vi "Controller Fast Command Loop.vi"(7 "Sync Objects":T1, 8 "error in (no error)":errorcluster, 11 "FOFB Configuration":T4={"FOFB Parameters"={"Network"={"FOFB Controller IP"="", "LNLS Control Network IP"="", "LNLS Control Network Power Supplies TCP Port"=0, "LNLS Control Network FOFB Configuration TCP Port"=0, "LNLS Control Network BPMs TCP Port"=0, "Monitoring Data TCP Port"=0, "Fast Archiver TCP Port"=0, "Fast Command TCP Port"=0, "TCP Listening Timeout"=0}, "Fast Acquisition"={"Sampling Period"=0, "Data Buffer Size"=0, "Monitoring Period"=0}, "Acquisition Network"=[], "Actuation Network"=[]}, "Number of Acquisition Chassis"=0, "Number of Actuation Chassis"=0, "Number of BPM Readings"=0, "BPM Reading Names"=[], "Selected BPM Readings"=[0, 1, 2, 3, 4, 5, 6, 7, 8, 9, 10, 11, 12, 13, 14, 15, 16, 17, 18, 19, 20, 21, 22, 23, 24, 25, 26, 27, 28, 29, 30, 31, 32, 33, 34, 35, 36, 37, 38, 39, 40, 41, 42, 43, 44, 45, 46, 47, 48, 49], "Number of Correctors"=0, "Corrector Names"=[], "Selected Correctors"=[0, 1, 2, 3, 4, 5, 6, 7, 8, 9, 10, 11, 12, 13, 14, 15, 16, 17, 18, 19, 20, 21, 22, 23, 24, 25, 26, 27, 28, 29, 30, 31, 32, 33, 34, 35, 36, 37, 38, 39, 40, 41, 42, 43, 44, 45, 46, 47, 48, 49], "Response Matrix"=[], "Reference Orbit"=[], "Correction Matrix"=[], "FPGA Filter Sets"=[], "Acquisition Chassis Names"=[], "Actuation Chassis Names"=[], "Acquisition Variables"=[], "Actuation Variables"=[], "PS Matrix Mapping"=[], "Inverse PS Matrix Mapping"=[], "BPM Matrix Mapping"=[], "Inverse BPM Matrix Mapping"=[], "BPM Planes"=[], "Corrector Planes"=[]}) -> (0 "error out":errorcluster)   [LabVIEW 2011]
uses:
  Types Definitions/Type FOFB Configuration.ctl
  Types Definitions/Type FOFB Parameters.ctl
  Types Definitions/Type Network Configuration.ctl
  Types Definitions/Type FA Configuration.ctl
  Types Definitions/Type Acquisition Network Configuration.ctl
  Types Definitions/Type Actuation Network Configuration.ctl
  Types Definitions/Type Synchronization Objects.ctl
  Types Definitions/Type Blocking Synchronization Objects.ctl
  Types Definitions/Type Monitoring Data.ctl
  Types Definitions/Type Operation Mode State.ctl
  Types Definitions/Type Diagnostics Data.ctl
  Types Definitions/Type CPU Loads Array.ctl
  Types Definitions/Type CPU Loads.ctl
  Types Definitions/Type Non-blocking Synchronization Objects.ctl
  Types Definitions/Type FOFB Variables.ctl
  Types Definitions/Type Actuation State.ctl
  Types Definitions/Type TCP State.ctl
  <vilib>/Platform/TimedLoop/XDataNode/timing_clust.ctl
  <vilib>/Platform/TimedLoop/XDataNode/nitl_modes.ctl
  <vilib>/Platform/TimedLoop/XDataNode/wakeup.ctl
  <vilib>/Platform/TimedLoop/XDataNode/XDataNode.xnode
  Type Definitions.lvlib
  <vilib>/Platform/TimedLoop/XDataNode/XDNodeRunTimeDep.lvlib
  Misc VIs.lvlib
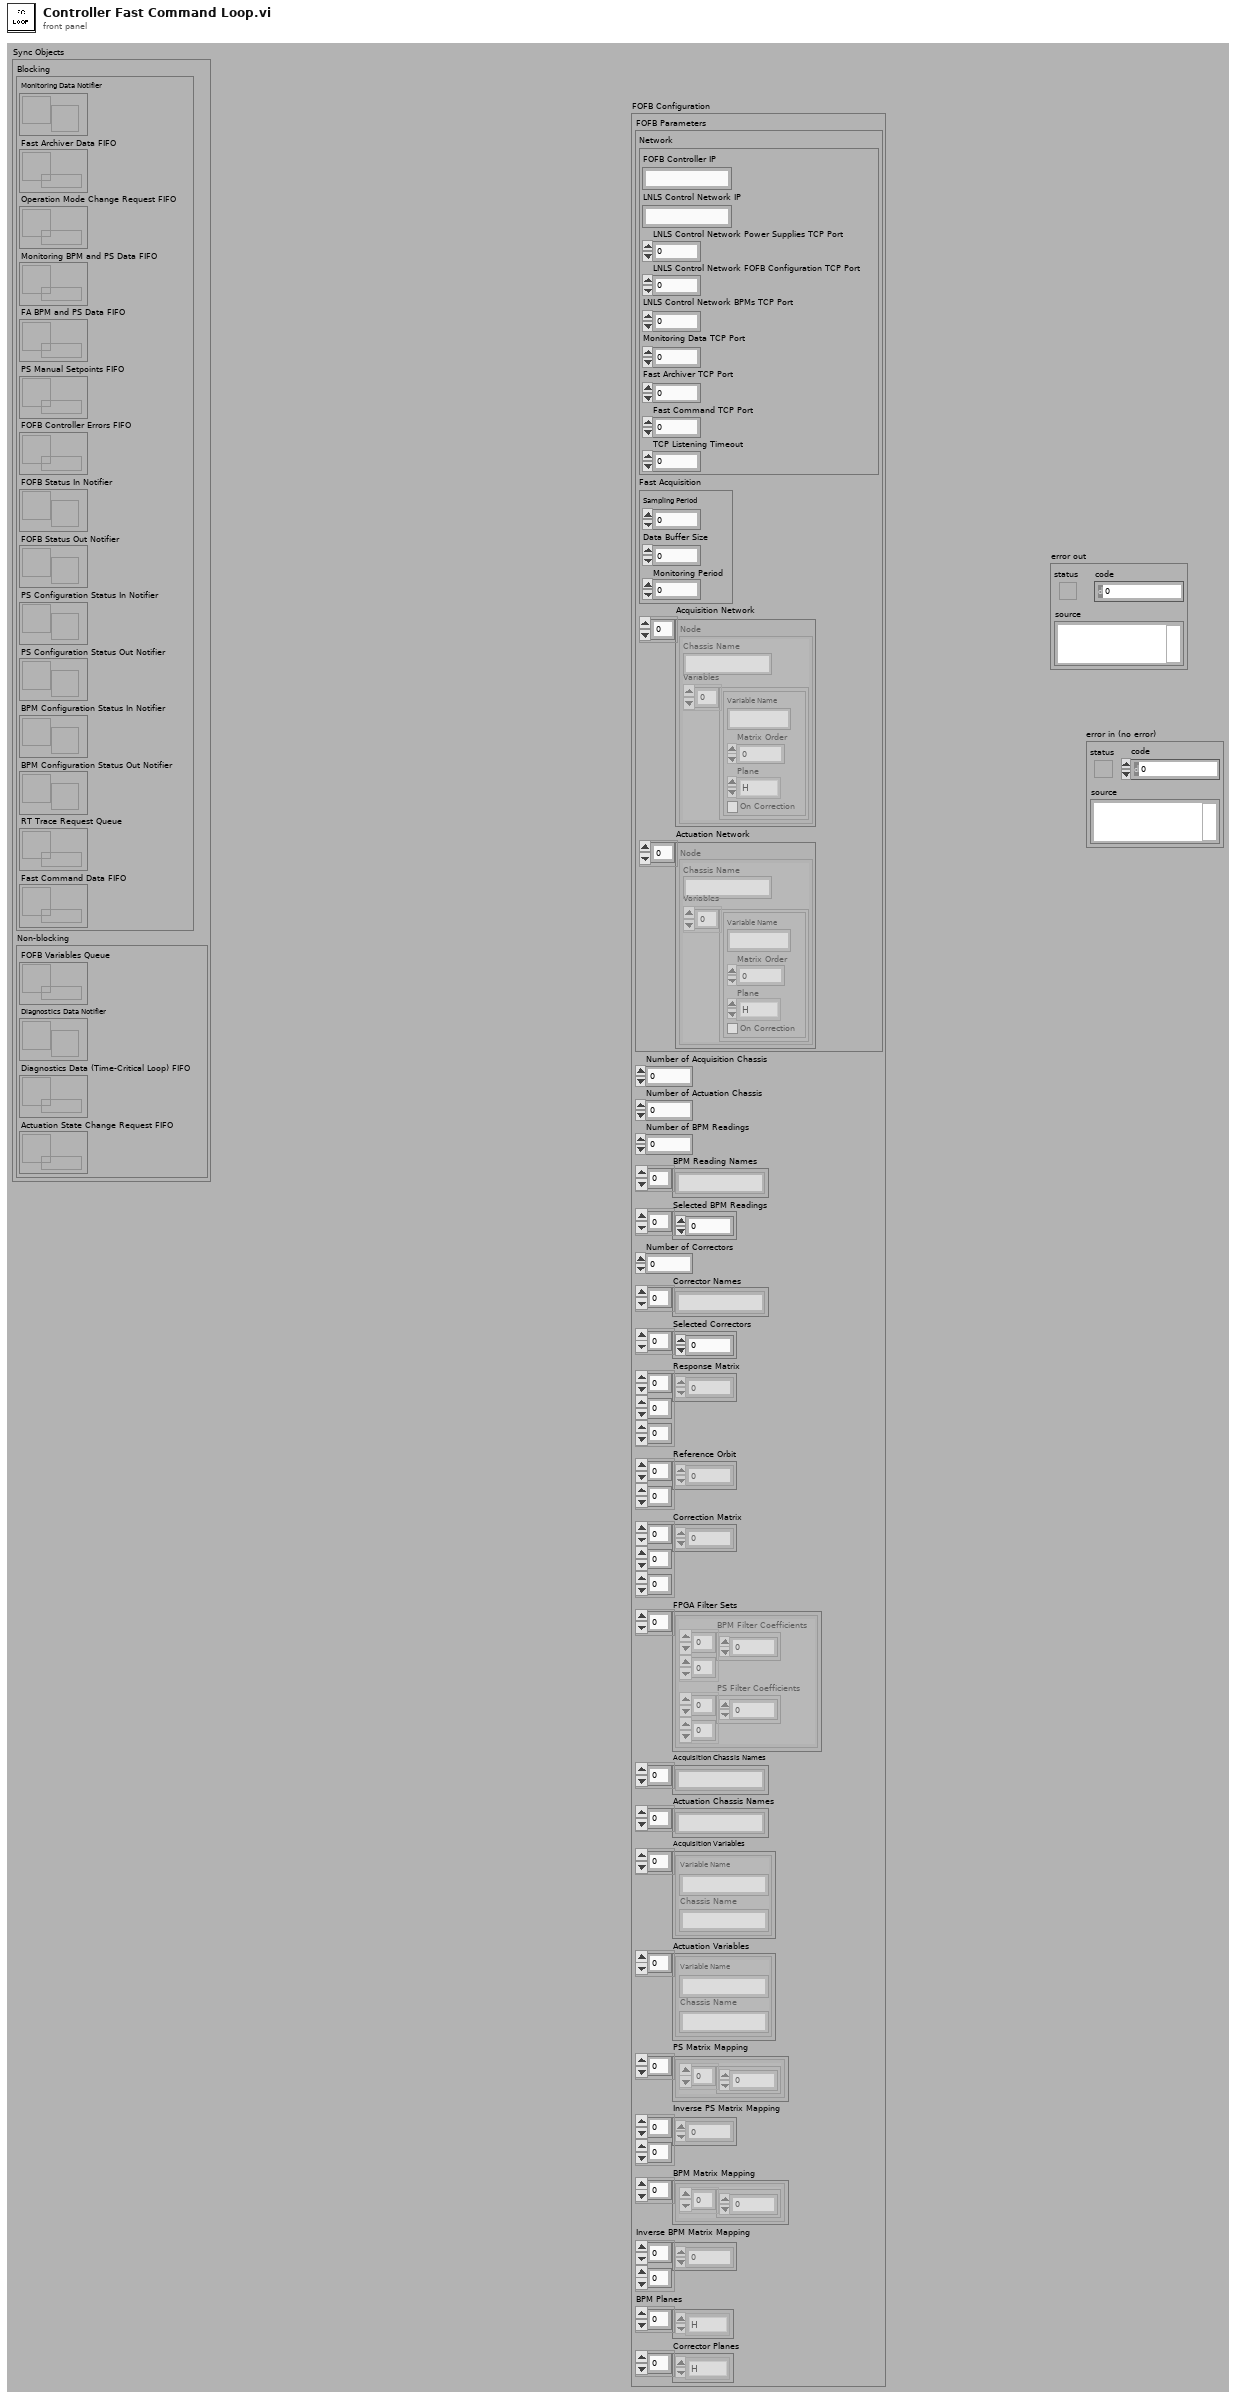
[diagram p1: front panel]
types:
  T1 = typedef "Type Definitions.lvlib/Type Synchronization Objects.ctl" = cluster{"Blocking":T2, "Non-blocking":T3}
  T2 = typedef "Type Definitions.lvlib/Type Blocking Synchronization Objects.ctl" = cluster{"Monitoring Data Notifier":refnum<notifier>, "Fast Archiver Data FIFO":refnum<queue>, "Operation Mode Change Request FIFO":refnum<k33>, "Monitoring BPM and PS Data FIFO":refnum<k33>, "FA BPM and PS Data FIFO":refnum<k33>, "PS Manual Setpoints FIFO":refnum<k33>, "FOFB Controller Errors FIFO ":refnum<k33>, "FOFB Status In Notifier":refnum<notifier>, "FOFB Status Out Notifier":refnum<notifier>, "PS Configuration Status In Notifier":refnum<notifier>, "PS Configuration Status Out Notifier":refnum<notifier>, "BPM Configuration Status In Notifier":refnum<notifier>, "BPM Configuration Status Out Notifier":refnum<notifier>, "RT Trace Request Queue":refnum<queue>, "Fast Command Data FIFO":refnum<k33>}
  T3 = typedef "Type Definitions.lvlib/Type Non-blocking Synchronization Objects.ctl" = cluster{"FOFB Variables Queue":refnum<queue>, "Diagnostics Data Notifier":refnum<notifier>, "Diagnostics Data (Time-Critical Loop) FIFO":refnum<k33>, "Actuation State Change Request FIFO":refnum<k33>}
  T4 = typedef "Type Definitions.lvlib/Type FOFB Configuration.ctl" = cluster{"FOFB Parameters":T5, "Number of Acquisition Chassis":i32, "Number of Actuation Chassis":i32, "Number of BPM Readings":i32, "BPM Reading Names":string[], "Selected BPM Readings":u32[], "Number of Correctors":i32, "Corrector Names":string[], "Selected Correctors":u32[], "Response Matrix":dbl[][][], "Reference Orbit":dbl[][], "Correction Matrix":dbl[][][], "FPGA Filter Sets":cluster{"BPM Filter Coefficients":dbl[][], "PS Filter Coefficients":dbl[][]}[], "Acquisition Chassis Names":string[], "Actuation Chassis Names":string[], "Acquisition Variables":cluster{"Variable Name":string, "Chassis Name":string}[], "Actuation Variables":cluster{"Variable Name":string, "Chassis Name":string}[], "PS Matrix Mapping":cluster{u32[]}[], "Inverse PS Matrix Mapping":u32[][], "BPM Matrix Mapping":cluster{u32[]}[], "Inverse BPM Matrix Mapping":u32[][], "BPM Planes":enum8{"H", "V"}[], "Corrector Planes":enum8{"H", "V"}[]}
  T5 = typedef "Type Definitions.lvlib/Type FOFB Parameters.ctl" = cluster{"Network":T6, "Fast Acquisition":T7, "Acquisition Network":T8, "Actuation Network":T9}
  T6 = typedef "Type Definitions.lvlib/Type Network Configuration.ctl" = cluster{"FOFB Controller IP":string, "LNLS Control Network IP":string, "LNLS Control Network Power Supplies TCP Port":u16, "LNLS Control Network FOFB Configuration TCP Port":u16, "LNLS Control Network BPMs TCP Port":u16, "Monitoring Data TCP Port":u16, "Fast Archiver TCP Port":u16, "Fast Command TCP Port":u16, "TCP Listening Timeout":i32}
  T7 = typedef "Type Definitions.lvlib/Type FA Configuration.ctl" = cluster{"Sampling Period":u32, "Data Buffer Size":u32, "Monitoring Period":u32}
  T8 = typedef "Type Definitions.lvlib/Type Acquisition Network Configuration.ctl" = cluster{"Chassis Name":string, "Variables":cluster{"Variable Name":string, "Matrix Order":u32, "Plane":enum8{"H", "V"}, "On Correction":bool}[]}[]
  T9 = typedef "Type Definitions.lvlib/Type Actuation Network Configuration.ctl" = cluster{"Chassis Name":string, "Variables":cluster{"Variable Name":string, "Matrix Order":u32, "Plane":enum8{"H", "V"}, "On Correction":bool}[]}[]
  T10 = enum16{"big-endian, network order", "native, host order", "little-endian"}
  T11 = typedef "Type Definitions.lvlib/Type TCP State.ctl" = enum16{"Idle", "Wait Connection", "Read Data", "Process Data", "Write Data", "Close Connection"}
  T12 = typedef "XDNodeRunTimeDep.lvlib/timing_clust.ctl" = cluster{"Expected End [f-1]":u64, "Actual End [f-1]":u64, "Finished Late? [f-1]":bool, "Expected End [i-1]":u64, "Actual End [i-1]":u64, "Finished Late? [i-1]":bool, "Expected Start [i]":u64, "Actual Start [i]":u64, "Expected Start [f]":u64, "Actual Start [f]":u64, "Source Name":string, "Structure Name":string, "Period":i64, "Deadline":i64, "Offset":i64, "Start":i64, "Priority":i32, "Timeout":i32, "Mode":T13, "Wakeup Reason":T14, "Error":errorcluster, "Source Type":string, "Secondary Source Type":string, "Global End Time":u64, "Global Start Time":u64, "Frame Duration":u64, "Iteration Duration":u64, "Assigned CPU":i32, "I/O Scan Engine Mode":u32}
  T13 = typedef "XDNodeRunTimeDep.lvlib/nitl_modes.ctl" = enum32{"No Change", "Process missed periods, maintain original phase", "Discard missed periods, maintain original phase", "Process missed periods, ignore original phase", "Discard missed periods, ignore original phase"}
  T14 = typedef "XDNodeRunTimeDep.lvlib/wakeup.ctl" = enum32{"Normal", "Aborted", "Asynchronous wakeup", "Timing source error", "Timed loop error", "Timeout"}
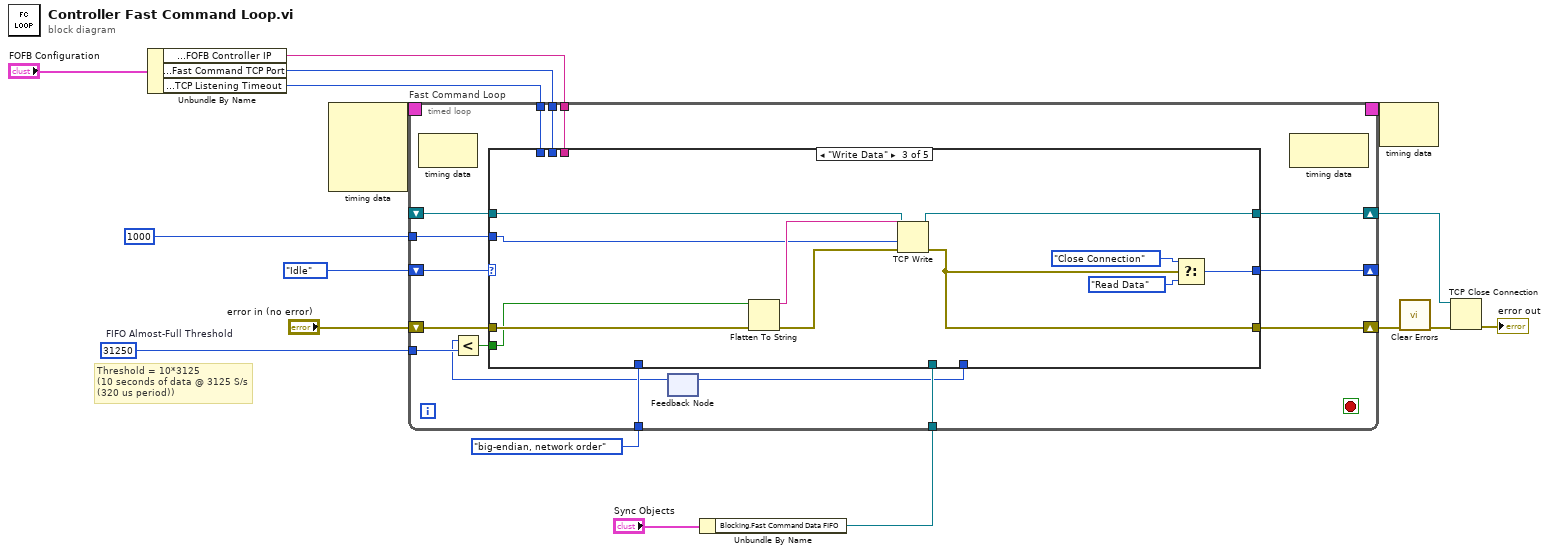
[diagram p0: block diagram]
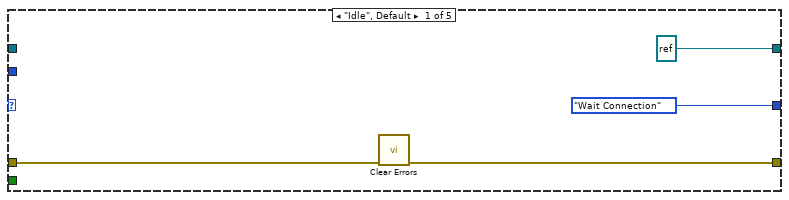
[diagram p2: hidden frame]
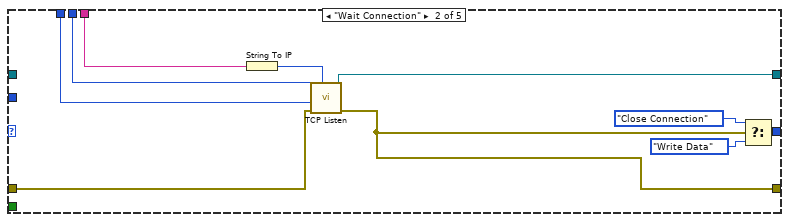
[diagram p3: hidden frame]
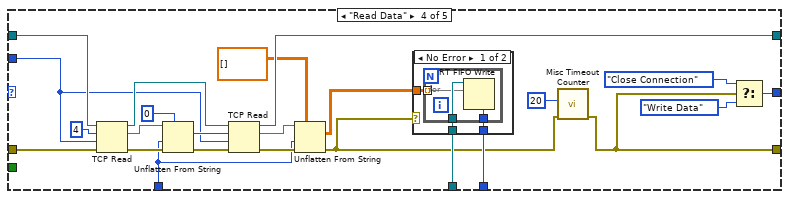
[diagram p4: hidden frame]
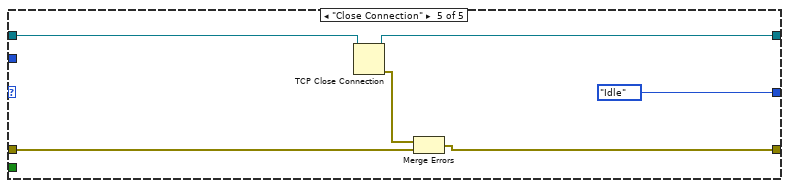
[diagram p6: hidden frame]
diagram:
  w11 = u32 31250  # FIFO Almost-Full Threshold
  # "Threshold = 10*3125\n(10 seconds of data @ 3125 S/s\n(320 us period))"
  n1 = Unbundle By Name("FOFB Configuration") -> ("FOFB Parameters.Network.FOFB Controller IP"=w5:string, "FOFB Parameters.Network.Fast Command TCP Port"=w3:u16, "FOFB Parameters.Network.TCP Listening Timeout"=w6:i32)
  n2 = node-c288() -> (w16:T12)  [unwired: 4 in]
  n3 = Unbundle By Name("Sync Objects") -> ("Blocking.Fast Command Data FIFO"=w4:refnum<k33>)
  n4 = timed-loop "Fast Command Loop" {
    tunnel: w5 -> [w33]
    tunnel: w3 -> [w32]
    tunnel: w6 -> [w31]
    shift-right: [w18] -> w10
    shift-left: "error in (no error)" -> [w26]
    shift-right: [w29] -> _
    shift-left: Type_TCP_State."Idle" ("f") -> [w30]
    shift-right: [w27] -> w12
    shift-left: _ -> [w28]
    timing: w16 -> [_]
    timing-out: [_] -> w15
    tunnel: T10."big-endian, network order" ("byte order (0:big-endian, network order)") -> [w25]
    tunnel: w4 -> [w24]
    tunnel: w11 -> [w23]
    tunnel: 1000 ("TCP Listening Timeout") -> [w19]
    stop <- _ stop-if-true
    n5 = node-c288() -> ()  [unwired: 1 in, 1 out]
    n6 = feedback #1() -> (w21:u32)  [unwired: 1 in]
    n7 = Less?(x=w21, y=w23) -> (x < y?=w20:bool)
    n8 = case shown="\"Write Data\"" w30 {
      tunnel: [refnum<k5> refnum ("connection ID") w49 w60 w77 w96] -> w27
      tunnel: [Type_TCP_State."Wait Connection" ("f") w48 w59 w73 Type_TCP_State."Idle" ("f")] -> w29
      tunnel: [w36 w40 w57 w62 w91] -> w18
      tunnel: w26 -> [w37 w45 w56 w76 w92]
      tunnel: w28 -> [_ _ w53 w79 w94]
      tunnel: w33 -> [_ w42 _ _ _]
      tunnel: w32 -> [_ w44 _ _ _]
      tunnel: w31 -> [_ w41 _ _ _]
      tunnel: w25 -> [_ _ _ w65 _]
      tunnel: w20 -> [_ _ w52 _ _]
      tunnel: w24 -> [_ _ _ w67 _]
      tunnel: [_ _ _ w66 _] -> w22
      tunnel: w19 -> [_ _ w50 w64 _]
      frame "Idle", Default {
        n9 = call <vilib>:"Clear Errors.vi"("error in (no error)"=w37) -> ("error out"=w36:errorcluster)  [unwired: 6 in]
      }
      frame "Wait Connection" {
        n10 = String To IP(1:w42) -> (0:w43:u32)
        n11 = call <vilib>:"TCP Listen.vi"("net address"=w43, "error in (no error)"=w45, "timeout ms (wait forever: -1)"=w41, "port"=w44) -> ("error out"=w40:errorcluster, "connection ID"=w49:refnum<k5>)  [unwired: 3 in, 3 out]
        n12 = Select(t=Type_TCP_State."Close Connection" ("f"), s=w40, f=Type_TCP_State."Write Data") -> (s? t:f=w48:T11)
      }
      frame "Write Data" {
        n13 = Flatten To String(anything=w52, error in (no error)=w56) -> (data string=w54:string, error out=w55:errorcluster)  [unwired: 2 in, 1 out]
        n14 = TCP Write(connection ID=w53, data in=w54, error in (no error)=w55, 9:w50) -> (connection ID out=w60:refnum<k5>, error out=w57:errorcluster)  [unwired: 1 out]
        n15 = Select(t=Type_TCP_State."Close Connection" ("f"), s=w57, f=Type_TCP_State."Read Data") -> (s? t:f=w59:T11)
      }
      frame "Read Data" {
        n16 = TCP Read(connection ID=w79, bytes to read=4, error in (no error)=w76, 9:w64) -> (connection ID out=w78:refnum<k5>, data out=w84:string, error out=w82:errorcluster)  [unwired: 1 in]
        n17 = Unflatten From String(type=0 ("length"), binary string=w84, byte order (0:big-endian, network order)=w65, error in (no error)=w82) -> (value=w69:i32, error out=w81:errorcluster)  [unwired: 1 in, 1 out]
        n18 = TCP Read(connection ID=w78, bytes to read=w69, error in (no error)=w81, 9:w64) -> (connection ID out=w77:refnum<k5>, data out=w68:string, error out=w80:errorcluster)  [unwired: 1 in]
        n19 = Unflatten From String(type=sgl[][] [], binary string=w68, byte order (0:big-endian, network order)=w65, error in (no error)=w80) -> (value=w71:sgl[][], error out=w63:errorcluster)  [unwired: 1 in, 1 out]
        n20 = case shown="No Error" w63 {
          tunnel: w71 -> [w87 _]
          tunnel: w67 -> [w86 _]
          tunnel: [w85 _] -> w66
          frame No Error {
            n21 = for {
              tunnel: w87 -> [w88] mode=indexing
              tunnel: w86 -> [w90]
              tunnel: [w89] -> w85
              n22 = RT FIFO Write(0:w90, 1:w88) -> (7:w89:u32)  [unwired: 3 in, 3 out]
            }
          }
          frame Error {
          }
        }
        n23 = call "Misc Timeout Counter.vi"("error in (no error)"=w63, "number of tries (3)"=20) -> ("error out"=w62:errorcluster)  [unwired: 9 in]
        n24 = Select(t=Type_TCP_State."Close Connection" ("f"), s=w62, f=Type_TCP_State."Write Data") -> (s? t:f=w73:T11)
      }
      frame "Close Connection" {
        n25 = TCP Close Connection(connection ID=w94) -> (connection ID out=w96:refnum<k5>, error out=w93:errorcluster)  [unwired: 2 in]
        n26 = Merge Errors(w93, w92) -> (w91:errorcluster)
      }
    }
    n27 = feedback-in #1(w22) -> ()
    n28 = node-c288() -> ()  [unwired: 1 in, 1 out]
  }
  n29 = node-c288(w15) -> ()  [unwired: 1 out]
  n30 = call <vilib>:"Clear Errors.vi"("error in (no error)"=w10) -> ("error out"=w9:errorcluster)  [unwired: 6 in]
  n31 = TCP Close Connection(connection ID=w12, error in (no error)=w9) -> (error out=→"error out":errorcluster)  [unwired: 1 in, 1 out]
